vi "runscenario process Conditions - Preprocess.vi"(7 "Connection Refnum":T3, 8 "error in (no error)":errorcluster, 9 "Run Filter (\"\")":string, 10 "Condition":T1, 11 "Condition Stack (empty)":T1[](array[typedef])) -> (0 "error out":errorcluster, 1 "new Run Filter":string, 2 "Condition out":T1, 3 "Condition Stack":T1[](array[typedef]), 5 "dup Connection Refnum":T3)   [LabVIEW 2011]
uses:
  server/database/Scenarios/Conditions/Condition Record.ctl
  server/database/Scenarios/Conditions/Condition Operators.ctl
  SI.LIB/ODBC/SQL Controls/Connection Refnum.ctl
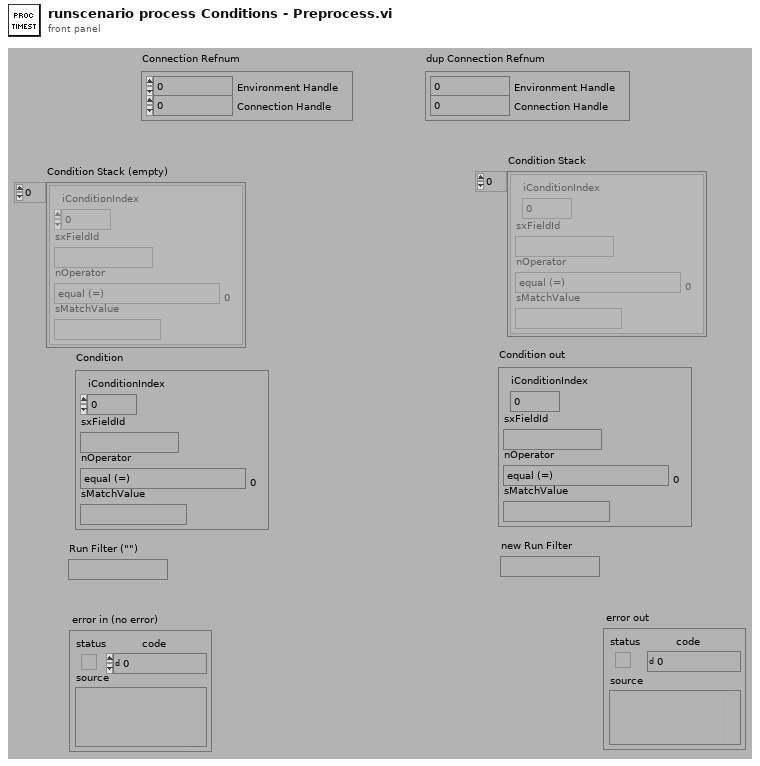
[diagram p1: front panel]
types:
  T1 = typedef "Condition Record.ctl" = cluster{"iConditionIndex":i32, "sxFieldId":string, "nOperator":T2, "sMatchValue":string}
  T2 = typedef "Condition Operators.ctl" = enum16{"equal (=)", "not equal (\\u2260)", "less than (<)", "less than or equal (\\u2264)", "greater than (>)", "greater than or equal (\\u2265)", "contains", "does not contain"}
  T3 = typedef "Connection Refnum.ctl" = cluster{"Environment Handle":i32, "Connection Handle":i32}
  T4 = typedef "Field Record.ctl" = cluster{"ixField":i32, "iSequenceOrder":i32, "sxFieldId":string, "sxSequenceId":string, "sDisplayName":string, "sValue":string, "sUnits":string, "nDataType":T5, "nNextItem":T6, "fSystem":bool, "fSystemValue":bool, "fRequired":bool, "fSetAtTest":bool, "fTestField":bool, "fDeleted":bool, "fIndexed":bool, "fFreeList":bool}
  T5 = typedef "Field DataTypes.ctl" = enum32{"text", "numeric", "list", "timestamp", "boolean"}
  T6 = typedef "Field NextItem.ctl" = enum32{"Reset", "Retain", "Auto-Increment"}
  T7 = cluster{"Day End":dbl, "Day Begin":dbl, "Day Prior Begin":dbl, "Week Begin":dbl, "Week Prior Begin":dbl, "Month Begin":dbl, "Month Prior Begin":dbl, "Year Begin":dbl, "Year Prior Begin":dbl}
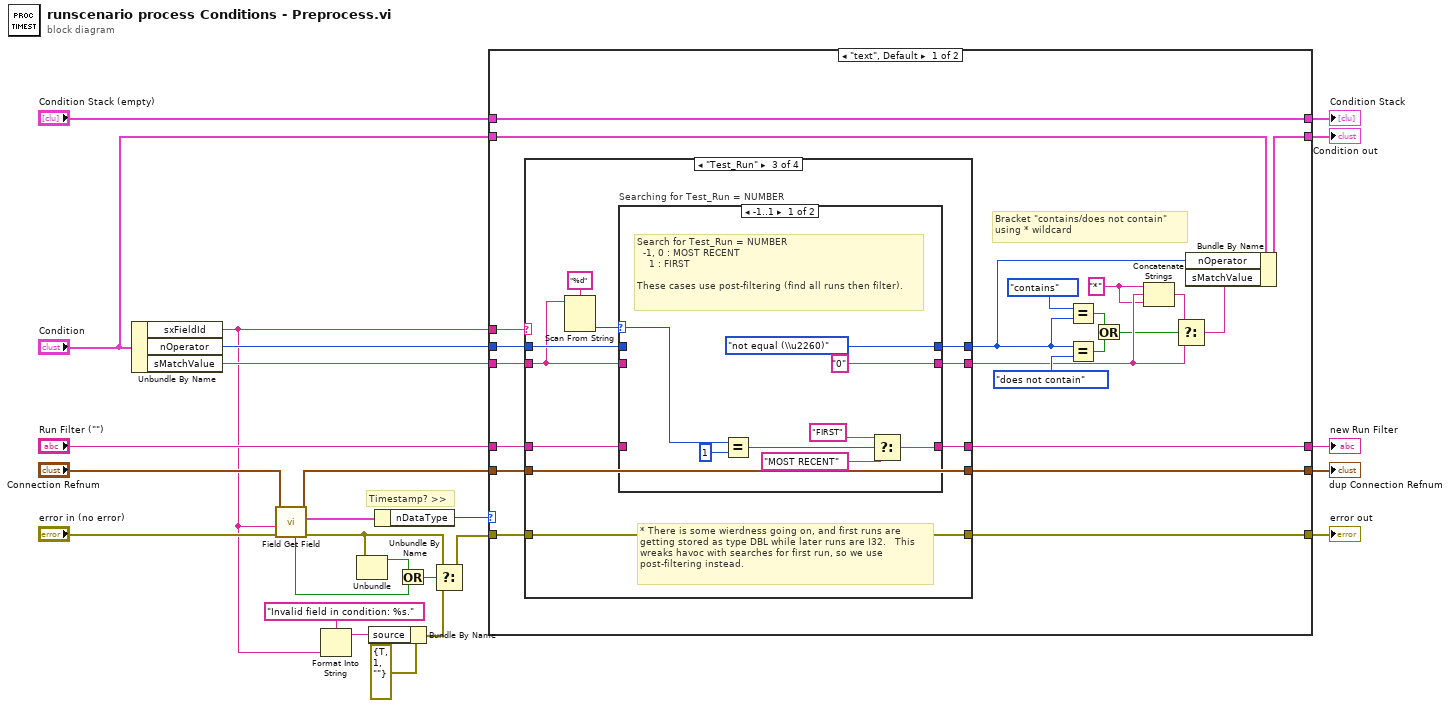
[diagram p0: block diagram]
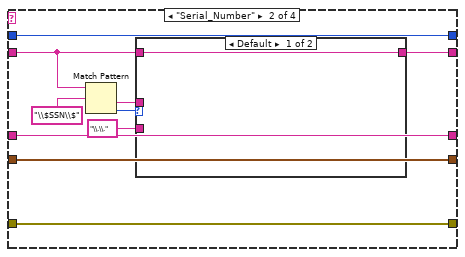
[diagram p3: hidden frame]
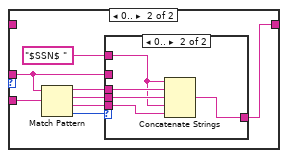
[diagram p4: hidden frame]
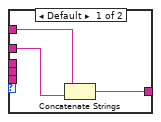
[diagram p5: hidden frame]
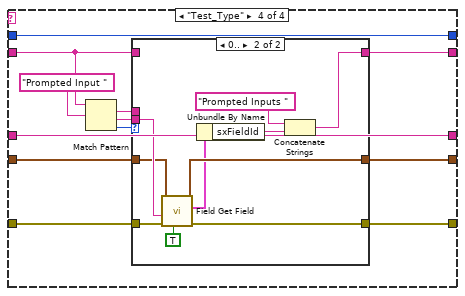
[diagram p7: hidden frame]
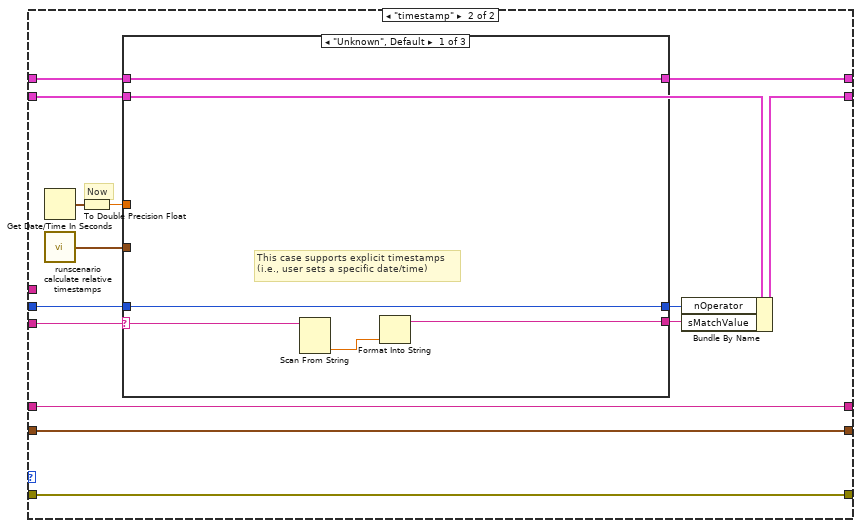
[diagram p9: hidden frame]
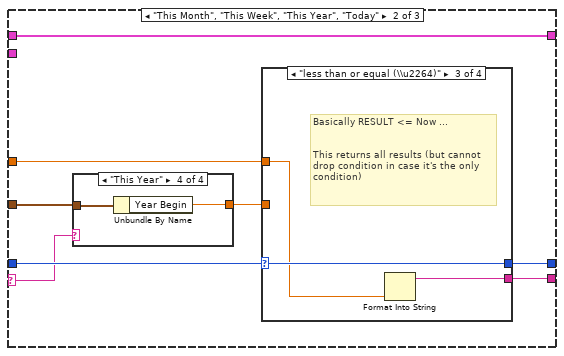
[diagram p10: hidden frame]
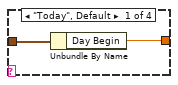
[diagram p11: hidden frame]
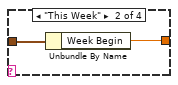
[diagram p12: hidden frame]
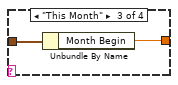
[diagram p13: hidden frame]
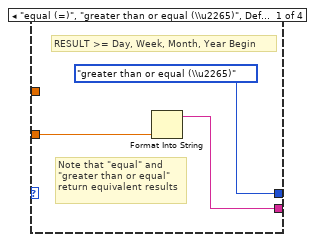
[diagram p14: hidden frame]
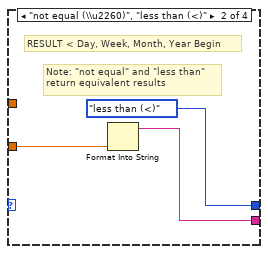
[diagram p15: hidden frame]
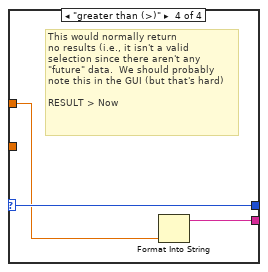
[diagram p16: hidden frame]
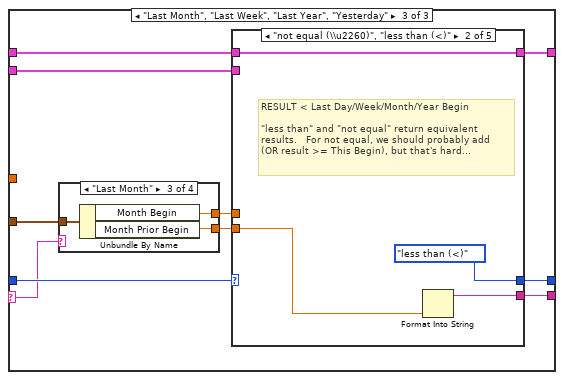
[diagram p17: hidden frame]
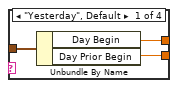
[diagram p18: hidden frame]
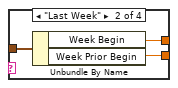
[diagram p19: hidden frame]
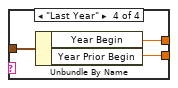
[diagram p20: hidden frame]
diagram:
  # "Timestamp? >>"
  n1 = Unbundle By Name("Condition") -> ("sxFieldId"=w5:string, "nOperator"=w15:T2, "sMatchValue"=w16:string)
  n2 = call "Field Get Field.vi"("error in (no error)"="error in (no error)", "sFieldId or sDisplayName (\"\")"=w5, "Connection Refnum"="Connection Refnum") -> ("error out"=w18:errorcluster, "Field"=w17:T4, "Connection Refnum"=w4:T3, "Data Present?"=w24:bool)  [unwired: 2 in, 3 out]
  n3 = Format Into String(format string="Invalid field in condition: %s." ("source"), w5) -> (resulting string=w20:string)  [unwired: 2 in, 1 out]
  n4 = Unbundle(w18) -> ("status"=w25:bool)  [unwired: 2 out]
  n5 = Bundle By Name(cluster=errorcluster {"status"=TRUE, "code"=1, "source"=""} ("error out"), "source"=w20) -> (w19:errorcluster)
  n6 = Unbundle By Name(w17) -> ("nDataType"=w10:T5)
  n7 = Or(x=w25, y=w24) -> (x .or. y?=w23:bool)
  n8 = Select(t=w18, s=w23, f=w19) -> (s? t:f=w3:errorcluster)
  n9 = case shown="\"text\", Default" w10 {
    tunnel: w16 -> [w35 w138]
    tunnel: w15 -> [w36 w139]
    tunnel: "Condition Stack (empty)" -> [w37 w137]
    tunnel: [w37 w136] -> w11
    tunnel: "Condition" -> [w34 w128]
    tunnel: "Run Filter (\"\")" -> [w39 w135]
    tunnel: [w38 w135] -> w7
    tunnel: [w31 w131] -> w6
    tunnel: w5 -> [w30 _]
    tunnel: w4 -> [w29 w126]
    tunnel: w3 -> [w28 w127]
    tunnel: [w27 w127] -> w2
    tunnel: [w26 w126] -> w1
    frame "text", Default {
      w40 = "*"
      # "Bracket \"contains/does not contain\"\nusing * wildcard"
      n10 = case shown="\"Test_Run\"" w30 {
        tunnel: [w50 w59 w83 w108] -> w46
        tunnel: w39 -> [w52 w62 w82 w111]
        tunnel: [w52 w62 w81 w111] -> w38
        tunnel: [w51 w55 w85 w112] -> w33
        tunnel: w36 -> [w51 w55 w86 w112]
        tunnel: w35 -> [w50 w56 w84 w107]
        tunnel: w29 -> [w49 w53 w88 w105]
        tunnel: w28 -> [w48 w54 w87 w104]
        tunnel: [w48 w54 w87 w103] -> w27
        tunnel: [w49 w53 w88 w102] -> w26
        frame "Default", Default {
        }
        frame "Serial_Number" {
          n11 = Match Pattern(string=w56, regular expression="\\$SSN\\$") -> (after substring=w58:string, offset past match=w60:i32)  [unwired: 3 out]
          n12 = case shown="Default" w60 {
            tunnel: [w63 w68] -> w59
            tunnel: w58 -> [_ w69]
            tunnel: "\\.\\." -> [_ w71]
            tunnel: w56 -> [w63 _]
            frame Default {
            }
            frame 0.. {
              n13 = Match Pattern(string=w69, regular expression=w71) -> (before substring=w67:string, match substring=w66:string, after substring=w65:string, offset past match=w70:i32)  [unwired: 1 out]
              n14 = case shown="0.." w70 {
                tunnel: w69 -> [w74 _]
                tunnel: [w73 w75] -> w68
                tunnel: "$SSN$ " -> [w72 w77]
                tunnel: w67 -> [_ w79]
                tunnel: w66 -> [_ w78]
                tunnel: w65 -> [_ w76]
                frame Default {
                  n15 = Concatenate Strings(w72, w74) -> (w73:string)
                }
                frame 0.. {
                  n16 = Concatenate Strings(w77, w79, w78, w77, w76) -> (w75:string)
                }
              }
            }
          }
        }
        frame "Test_Run" {
          # "* There is some wierdness going on, and first runs are\ngetting stored as type DBL while later runs are I32.   This\nwreaks havoc with searches for first run, so we use\npost-filtering instead."
          n17 = Scan From String(format string="%d" ("y"), input string=w84) -> (output 1=w80:i32)  [unwired: 2 in, 4 out]
          n18 = case "Searching for Test_Run = NUMBER" shown="-1..1" w80 {
            selector: w80 -> [w93 _]
            tunnel: w86 -> [_ w100]
            tunnel: [Condition_Operators."not equal (\\u2260)" ("y") w100] -> w85
            tunnel: w84 -> [_ w99]
            tunnel: ["0" ("y") w99] -> w83
            tunnel: w82 -> [_ w98]
            tunnel: [w91 w98] -> w81
            frame -1..1 {
              # "Search for Test_Run = NUMBER\n  -1, 0 : MOST RECENT\n    1 : FIRST\n\nThese cases use post-filtering (find all runs then filter)."
              n19 = Equal?(x=w93, y=1) -> (x = y?=w94:bool)
              n20 = Select(t="FIRST" ("y"), s=w94, f="MOST RECENT" ("y")) -> (s? t:f=w91:string)
            }
            frame 2.., Default {
              # "Search for Test_Run = NUMBER (2 or greater)..."
            }
          }
        }
        frame "Test_Type" {
          n21 = Match Pattern(string=w107, regular expression="Prompted Input ") -> (match substring=w101:string, after substring=w106:string, offset past match=w109:i32)  [unwired: 1 in, 1 out]
          n22 = case shown="0.." w109 {
            tunnel: [w115 w118] -> w108
            tunnel: w107 -> [w115 _]
            tunnel: w106 -> [_ w125]
            tunnel: w105 -> [w114 w124]
            tunnel: w104 -> [w113 w123]
            tunnel: [w113 w121] -> w103
            tunnel: [w114 w122] -> w102
            tunnel: w101 -> [_ _]
            frame Default {
            }
            frame 0.. {
              n23 = call "Field Get Field.vi"("by sDisplayName? (f, by sFieldId)"=TRUE, "error in (no error)"=w123, "sFieldId or sDisplayName (\"\")"=w125, "Connection Refnum"=w124) -> ("error out"=w121:errorcluster, "Field"=w120:T4, "Connection Refnum"=w122:T3)  [unwired: 1 in, 4 out]
              n24 = Unbundle By Name(w120) -> ("sxFieldId"=w119:string)
              n25 = Concatenate Strings("Prompted Inputs " ("regular expression"), w119) -> (w118:string)
            }
          }
        }
      }
      n26 = Equal?(x=Condition_Operators."contains" ("y"), y=w33) -> (x = y?=w41:bool)
      n27 = Equal?(x=w33, y=Condition_Operators."does not contain") -> (x = y?=w42:bool)
      n28 = Or(x=w41, y=w42) -> (x .or. y?=w43:bool)
      n29 = Concatenate Strings(w40, w46, w40) -> (w45:string)
      n30 = Select(t=w45, s=w43, f=w46) -> (s? t:f=w32:string)
      n31 = Bundle By Name(cluster=w34, "nOperator"=w33, "sMatchValue"=w32) -> (w31:T1)
    }
    frame "timestamp" {
      # "Now"
      n32 = Get Date/Time In Seconds() -> (seconds since 1Jan1904=w134:timestamp)
      n33 = call "runscenario calculate relative timestamps.vi"() -> ("UTC Relative Timestamps"=w132:T7)  [unwired: 1 in]
      n34 = To Double Precision Float(number=w134) -> (double precision float=w133:dbl)
      n35 = case shown="\"Unknown\", Default" w138 {
        selector: w138 -> [w142 w147 w173]
        tunnel: w139 -> [w143 w152 w182]
        tunnel: w137 -> [w144 w145 w181]
        tunnel: [w144 w145 w179] -> w136
        tunnel: [w143 w151 w180] -> w129
        tunnel: [w141 w150 w178] -> w130
        tunnel: w132 -> [_ w148 w175]
        tunnel: w133 -> [_ w149 _]
        tunnel: w128 -> [_ _ w177]
        frame "Unknown", Default {
          # "This case supports explicit timestamps\n(i.e., user sets a specific date/time)"
          n36 = Scan From String(input string=w142) -> (output 1=w140:dbl)  [unwired: 3 in, 4 out]
          n37 = Format Into String(w140) -> (resulting string=w141:string)  [unwired: 3 in, 1 out]
        }
        frame "This Month", "This Week", "This Year", "Today" {
          n38 = case shown="\"This Year\"" w147 {
            tunnel: w148 -> [w154 w156 w158 w160]
            tunnel: [w153 w155 w157 w159] -> w146
            frame "Today", Default {
              n39 = Unbundle By Name(w154) -> ("Day Begin"=w153:dbl)
            }
            frame "This Week" {
              n40 = Unbundle By Name(w156) -> ("Week Begin"=w155:dbl)
            }
            frame "This Month" {
              n41 = Unbundle By Name(w158) -> ("Month Begin"=w157:dbl)
            }
            frame "This Year" {
              n42 = Unbundle By Name(w160) -> ("Year Begin"=w159:dbl)
            }
          }
          n43 = case shown="\"less than or equal (\\\\u2264)\"" w152 {
            selector: w152 -> [_ _ w169 w172]
            tunnel: [Condition_Operators."greater than or equal (\\u2265)" ("nOperator") Condition_Operators."less than (<)" ("nOperator") w169 w172] -> w151
            tunnel: [w162 w165 w167 w170] -> w150
            tunnel: w149 -> [_ _ w168 w171]
            tunnel: w146 -> [w161 w164 _ _]
            frame "equal (=)", "greater than or equal (\\u2265)", Default {
              # "Note that \"equal\" and\n\"greater than or equal\"\nreturn equivalent results"
              # "RESULT >= Day, Week, Month, Year Begin"
              n44 = Format Into String(w161) -> (resulting string=w162:string)  [unwired: 3 in, 1 out]
            }
            frame "not equal (\\u2260)", "less than (<)" {
              # "Note: \"not equal\" and \"less than\"\nreturn equivalent results"
              # "RESULT < Day, Week, Month, Year Begin"
              n45 = Format Into String(w164) -> (resulting string=w165:string)  [unwired: 3 in, 1 out]
            }
            frame "less than or equal (\\u2264)" {
              # "Basically RESULT <= Now ...\n\n\nThis returns all results (but cannot \ndrop condition in case it's the only\ncondition)"
              n46 = Format Into String(w168) -> (resulting string=w167:string)  [unwired: 3 in, 1 out]
            }
            frame "greater than (>)" {
              # "This would normally return\nno results (i.e., it isn't a valid\nselection since there aren't any\n\"future\" data.  We should probably\nnote this in the GUI (but that's hard)\n\nRESULT > Now"
              n47 = Format Into String(w171) -> (resulting string=w170:string)  [unwired: 3 in, 1 out]
            }
          }
        }
        frame "Last Month", "Last Week", "Last Year", "Yesterday" {
          n48 = case shown="\"Last Month\"" w173 {
            tunnel: w175 -> [w185 w188 w191 w194]
            tunnel: [w184 w186 w189 w192] -> w176
            tunnel: [w183 w187 w190 w193] -> w174
            frame "Yesterday", Default {
              n49 = Unbundle By Name(w185) -> ("Day Begin"=w184:dbl, "Day Prior Begin"=w183:dbl)
            }
            frame "Last Week" {
              n50 = Unbundle By Name(w188) -> ("Week Begin"=w186:dbl, "Week Prior Begin"=w187:dbl)
            }
            frame "Last Month" {
              n51 = Unbundle By Name(w191) -> ("Month Begin"=w189:dbl, "Month Prior Begin"=w190:dbl)
            }
            frame "Last Year" {
              n52 = Unbundle By Name(w194) -> ("Year Begin"=w192:dbl, "Year Prior Begin"=w193:dbl)
            }
          }
          n53 = case shown="\"not equal (\\\\u2260)\", \"less than (<)\"" w182 {
            selector: w182 -> [_ _ w210 w214 w218]
            tunnel: w181 -> [w203 w206 w211 w215 w219]
            tunnel: [Condition_Operators."greater than or equal (\\u2265)" ("nOperator") Condition_Operators."less than (<)" ("nOperator") w210 w214 w218] -> w180
            tunnel: [w202 w206 w211 w215 w219] -> w179
            tunnel: [w199 w207 w212 w216 w220] -> w178
            tunnel: w177 -> [w198 _ _ _ _]
            tunnel: w176 -> [w196 _ w209 w213 _]
            tunnel: w174 -> [w195 w205 _ _ w217]
            frame "equal (=)", Default {
              # "RESULT < (this) Day/Week/Month/Year Begin\n\n   AND\n\nRESULT >= Last Day/Week/Month/Year Begin"
              n54 = Format Into String(w196) -> (resulting string=w200:string)  [unwired: 3 in, 1 out]
              n55 = Format Into String(w195) -> (resulting string=w199:string)  [unwired: 3 in, 1 out]
              n56 = Bundle By Name(cluster=w198, "nOperator"=Condition_Operators."less than (<)", "sMatchValue"=w200) -> (w197:T1)
              n57 = Build Array (concatenate)(w203, w197) -> (w202:T1[])
            }
            frame "not equal (\\u2260)", "less than (<)" {
              # "RESULT < Last Day/Week/Month/Year Begin\n\n\"less than\" and \"not equal\" return equivalent\nresults.   For not equal, we should probably add \n(OR result >= This Begin), but that's hard..."
              n58 = Format Into String(w205) -> (resulting string=w207:string)  [unwired: 3 in, 1 out]
            }
            frame "less than or equal (\\u2264)" {
              # "RESULT <= (this) day/week/month/year begin"
              n59 = Format Into String(w209) -> (resulting string=w212:string)  [unwired: 3 in, 1 out]
            }
            frame "greater than (>)" {
              # "RESULT > (this) day/week/month/year Begin"
              n60 = Format Into String(w213) -> (resulting string=w216:string)  [unwired: 3 in, 1 out]
            }
            frame "greater than or equal (\\u2265)" {
              # "result >= Yesterday, Last Week/Month/Year Begin"
              n61 = Format Into String(w217) -> (resulting string=w220:string)  [unwired: 3 in, 1 out]
            }
          }
        }
      }
      n62 = Bundle By Name(cluster=w128, "nOperator"=w129, "sMatchValue"=w130) -> (w131:T1)
    }
  }
  "error out" <- w2
  "Condition Stack" <- w11
  "dup Connection Refnum" <- w1
  "Condition out" <- w6
  "new Run Filter" <- w7
